vi "Frame.Export.StringArray.vi"(8 "error in (no error)":errorcluster, 11 "Frame Parameters":T1[](array[typedef]) {"Byte Order" items=["Little Endian", "Big Endian"]; "Data Type" items=["Signed", "Unsigned", "IEEE Float"]}) -> (0 "error out":errorcluster, 3 "Frame Parameters":string[][](array[string]))   [LabVIEW 2019, in "Diagnostics Addon System Explorer.lvlib"]
uses:
  Diagnostics Addon System Explorer.lvlib
  Addon Shared/Types/Signal.ctl
  Addon Shared/Diagnostics Addon Shared.lvlib
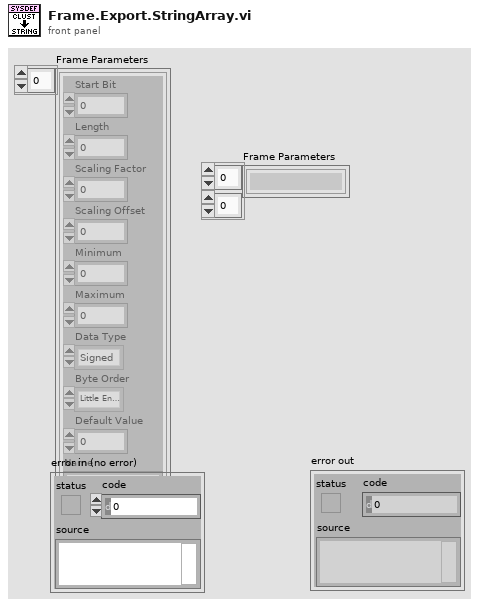
[diagram p1: front panel]
types:
  T1 = typedef "Diagnostics Addon Shared.lvlib/Signal.ctl" = cluster{"Start Bit":u32, "Length":u32, "Scaling Factor":dbl, "Scaling Offset":dbl, "Minimum":dbl, "Maximum":dbl, "Data Type":u32, "Byte Order":u32, "Default Value":dbl, "Name":string, "Units":string}
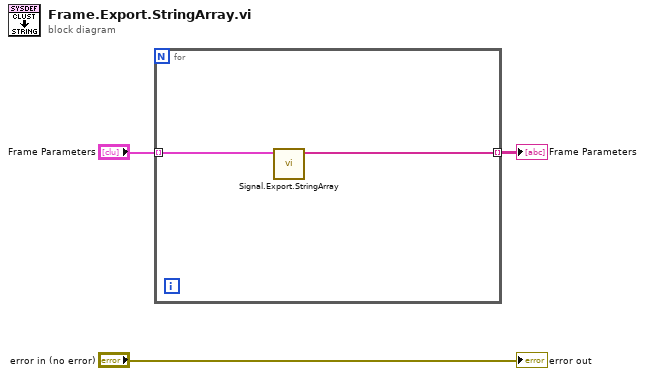
[diagram p0: block diagram]
diagram:
  n1 = for {
    tunnel: [w5] -> w3 mode=indexing
    tunnel: "Frame Parameters" -> [w4] mode=indexing
    n2 = call "Signal.Export.StringArray.vi"("Signal Parameters"=w4) -> ("Array"=w5:string[])  [unwired: 10 in]
  }
  "Frame Parameters" <- w3
  "error out" <- "error in (no error)"
